vi "Autonomous Independent.vi"() -> ()   [LabVIEW 2020]
doc: "This VI is called when autonomous begins, and will automatically be terminated when autonomous ends. You can carry out timed or sensor driven robot movement independently without needing to return to the caller."
uses:
  <vilib>/Rock Robotics/WPI/RobotDrive/WPI_RobotDriveArcadeDrive_Standard(NoSaturation).vi
  <vilib>/Rock Robotics/Network Tables/NT Write Numeric Array.vi
  <vilib>/Rock Robotics/Network Tables/NT Read String.vi
panel:
  in  "Array for intake":cluster{"Delay (sec)":dbl, "On or Off":bool}[](array[cluster])
  out "Current Movement, for debugging":T1 {"Y Joystick Value" scale=1.0..-1.0; "X Joystick Value" scale=-1.0..1.0}
  in  "Array of robot movements":T2(array[cluster])=[{"X Joystick Value"=0.39393939393939403, "Y Joystick Value"=0.0, "Delay (sec)"=1.0, "Movement Name"="turn"}, {"X Joystick Value"=-0.3737373737373737, "Y Joystick Value"=0.0, "Delay (sec)"=1.0, "Movement Name"="turn back"}] {"Y Joystick Value" scale=1.0..-1.0; "X Joystick Value" scale=-1.0..1.0}
  # "Be sure to right-click and choose Data Operations>>Make Current Value default if you want to save the array values with the VI"
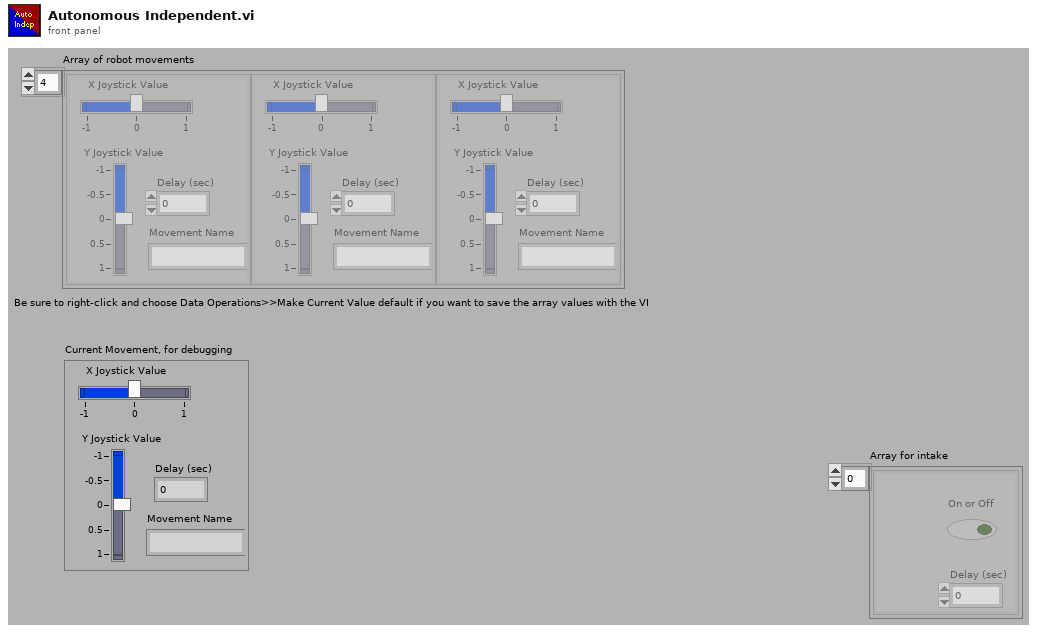
[diagram p1: front panel]
types:
  T1 = cluster{"X Joystick Value":dbl, "Y Joystick Value":dbl, "Delay (sec)":dbl, "Movement Name":string}
  T2 = cluster{"X Joystick Value":dbl, "Y Joystick Value":dbl, "Delay (sec)":dbl, "Movement Name":string}[]
  T3 = typedef "WPI_JoystickDevRef.ctl" = cluster{"Device":T4}
  T4 = typedef "WPI_JoystickDeviceEnum.ctl" = enum16{"USB 0", "USB 1", "USB 2", "USB 3", "USB 4", "USB 5"}
  T5 = typedef "WPI_MotorControlDeviceRef.ctl" = cluster{"DeviceStatus":errorcluster, "Type":T6, "PWM":cluster{"PWM Channel":T7, "DeadBand":T8}, "CAN":cluster{"Device Number":u8, "SetOutput VI Ref":variant, "GetOutput VI Ref":variant, "Enable VI Ref":variant, "Disable VI Ref":variant, "Data":variant}, "Invert":bool, "DIO PWM":cluster{"PWM \"Enable\" Channel":T7, "DIOChannel":T9, "PWM Rate":dbl}}
  T6 = typedef "WPI_MotorControlType.ctl" = enum16{"PWM", "CAN", "DIO PWM"}
  T7 = typedef "FPGA_DIOPWMChannel.ctl" = enum8{"PWM 0", "PWM 1", "PWM 2", "PWM 3", "PWM 4", "PWM 5", "PWM 6", "PWM 7", "PWM 8", "PWM 9", "PWM MXP 0", "PWM MXP 1", "PWM MXP 2", "PWM MXP 3", "PWM MXP 4", "PWM MXP 5", "PWM MXP 6", "PWM MXP 7", "PWM MXP 8", "PWM MXP 9", "Invalid"}
  T8 = typedef "WPI_PWMDeadband.ctl" = cluster{"Name":string, "maxPositivePwm":i32, "minPositivePwm":i32, "centerPwm":i32, "maxNegativePwm":i32, "minNegativePwm":i32, "angularRange":u16}
  T9 = typedef "FPGA_DIOChannel.ctl" = enum8{"DIO 0", "DIO 1", "DIO 2", "DIO 3", "DIO 4", "DIO 5", "DIO 6", "DIO 7", "DIO 8", "DIO 9", "DIO MXP 0", "DIO MXP 1", "DIO MXP 2", "DIO MXP 3", "DIO MXP 4", "DIO MXP 5", "DIO MXP 6", "DIO MXP 7", "DIO MXP 8", "DIO MXP 9", "DIO MXP 10", "DIO MXP 11", "DIO MXP 12", "DIO MXP 13", "DIO MXP 14", "DIO MXP 15", "SPI Port CS1", "SPI Port CS2", "SPI Port CS3", "SPI Port MISO", "SPI Port MOSI", "Invalid"}
  T10 = typedef "WPI_RobotDriveDevRef.ctl" = cluster{"DevStatus":errorcluster, "Motors[]":T5[], "Square Inputs":bool, "Max Output":dbl}
  T11 = cluster{"Yaw":dbl, "Roll":dbl, "Pitch":dbl, "Heading":dbl, "Fused Heading":dbl}
  T12 = typedef "Color Sensor V3 DevRef.ctl" = cluster{"I2CDevRef":T13}
  T13 = typedef "WPI_I2CDevRef.ctl" = cluster{"DevStatus":errorcluster, "Device Address":u8, "Handle":i32, "I2C Bus":T14}
  T14 = typedef "i2c_bus.ctl" = enum16{"I2C On-Board", "I2C MXP", "Invalid"}
  T15 = typedef "WPI_SwitchDevRef.ctl" = cluster{"DevStatus":errorcluster, "DIO Channel":T9, "CntIndex":T16, "Normally Closed":bool}
  T16 = typedef "FPGA_CounterCtrSystemIndex.ctl" = enum8{"Ctr 0", "Ctr 1", "Ctr 2", "Ctr 3", "Ctr 4", "Ctr 5", "Ctr 6", "Ctr 7", "Invalid"}
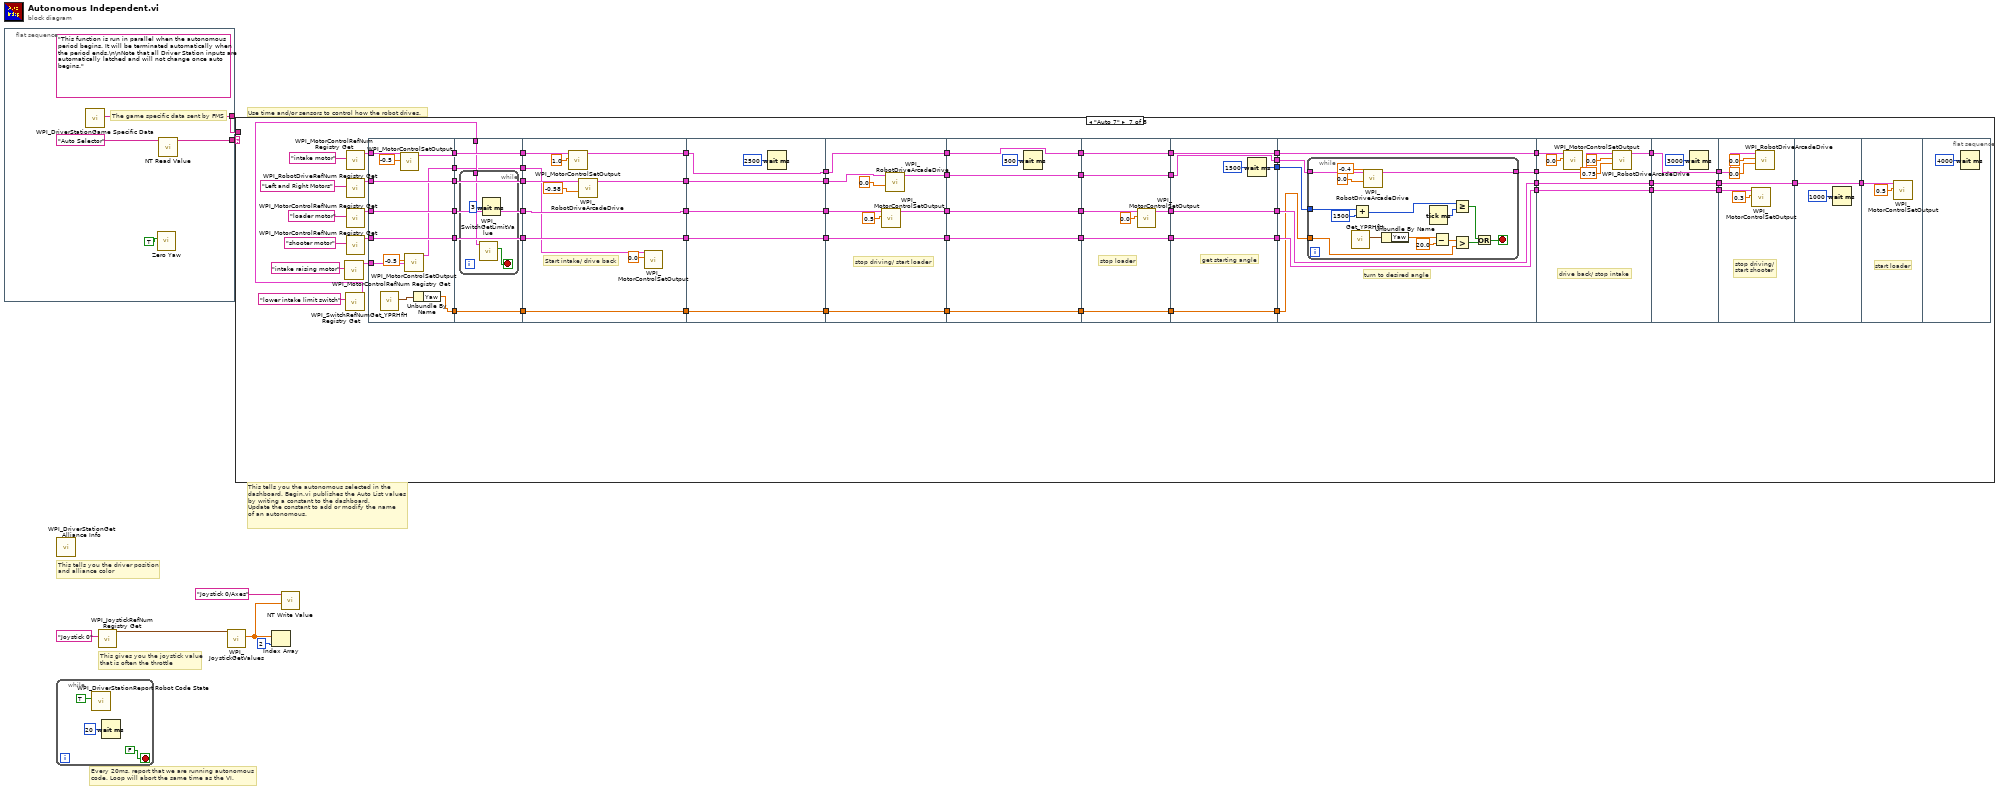
[diagram p0: block diagram]
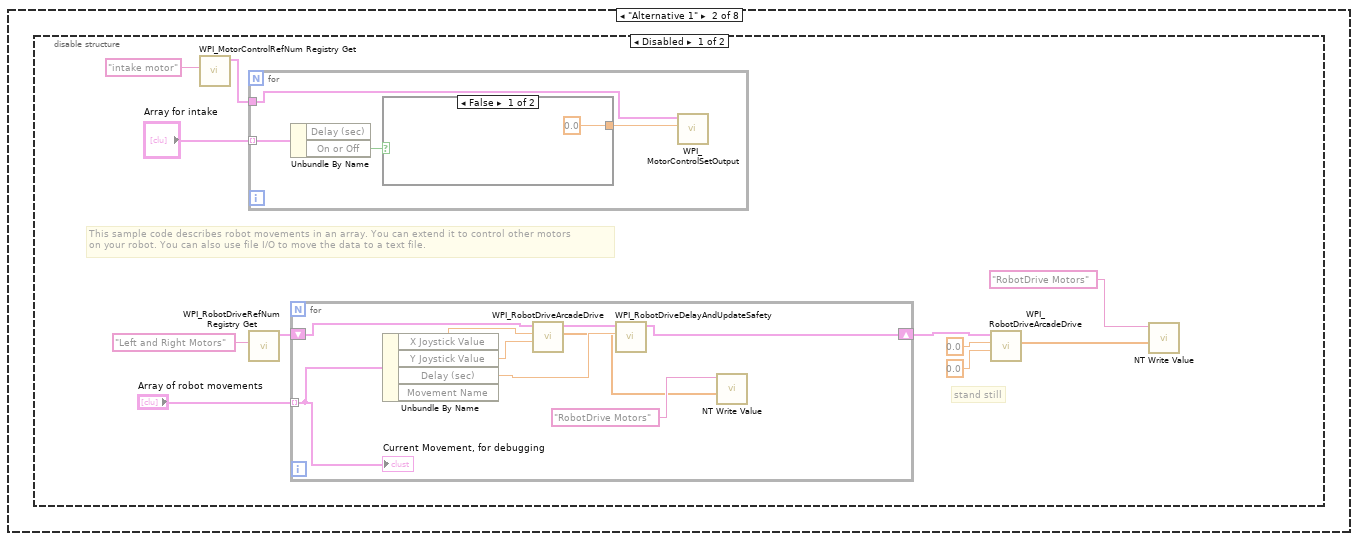
[diagram p3: hidden frame]
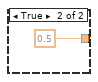
[diagram p4: hidden frame]
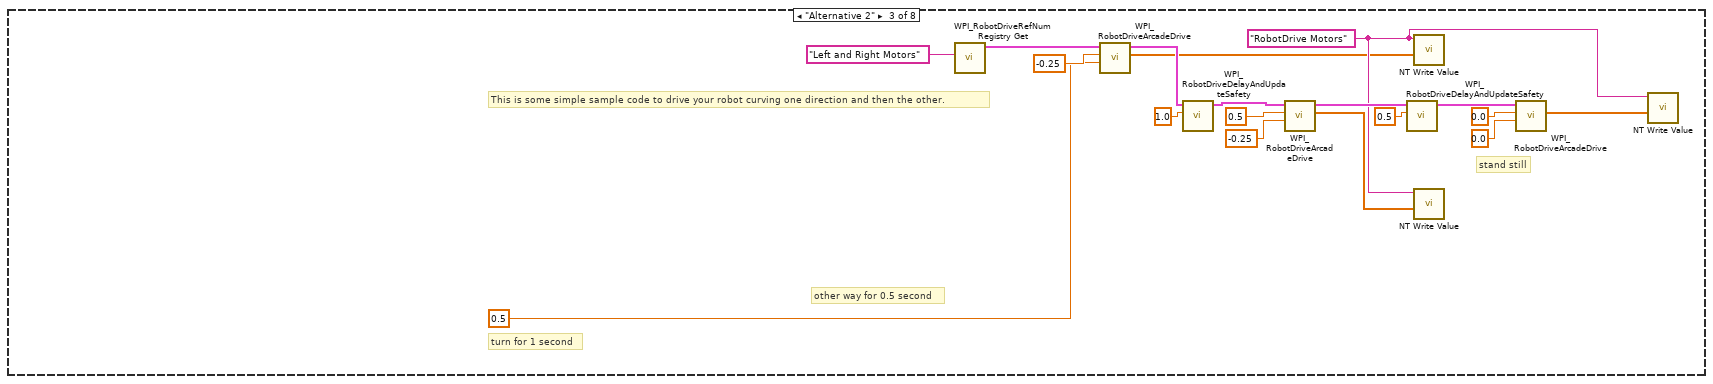
[diagram p6: hidden frame]
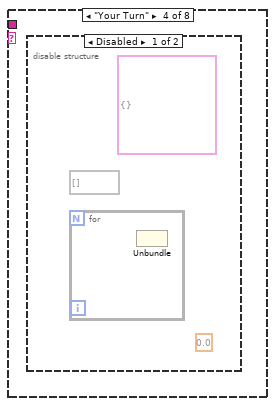
[diagram p7: hidden frame]
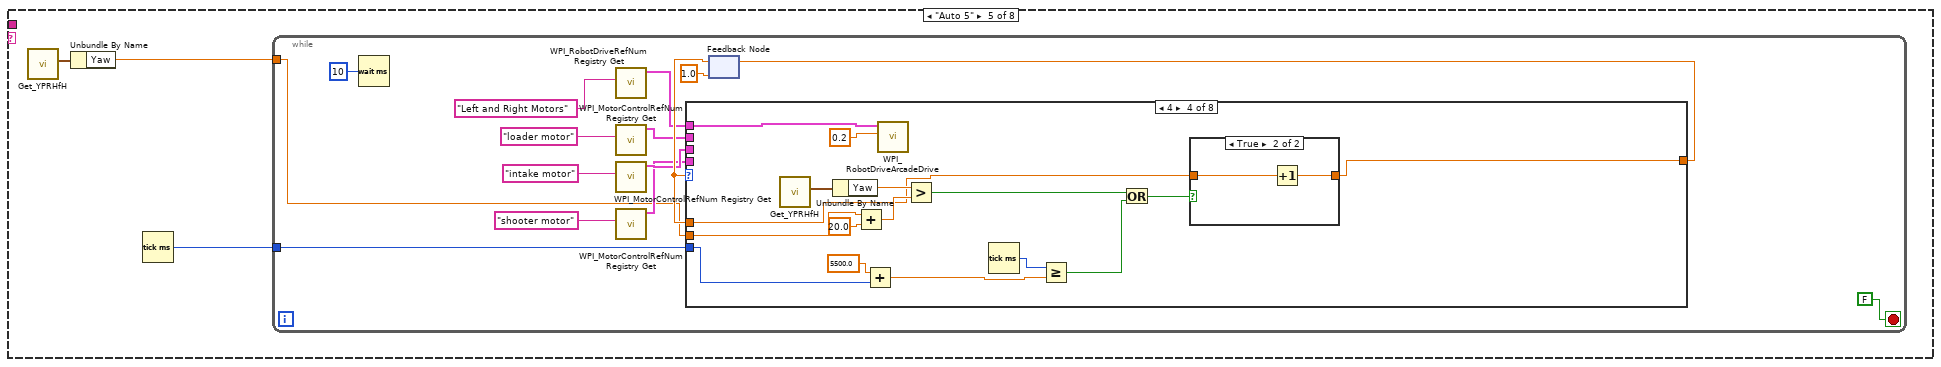
[diagram p9: hidden frame]
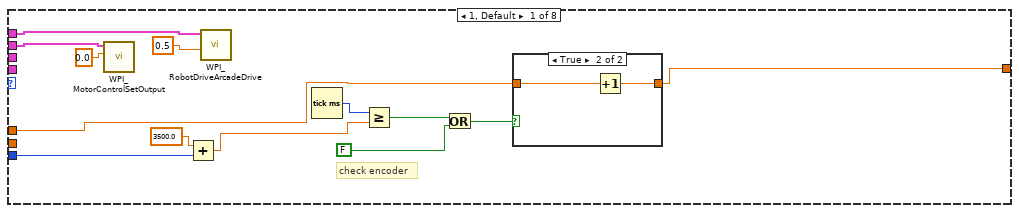
[diagram p10: hidden frame]
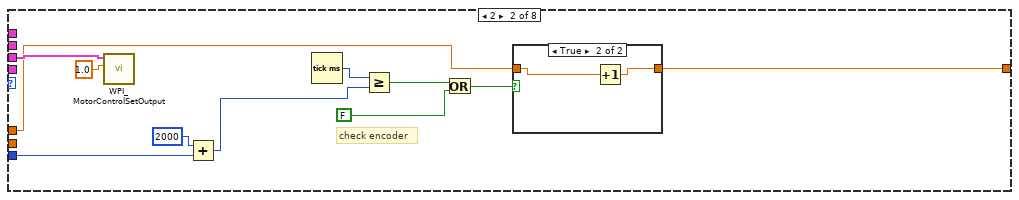
[diagram p12: hidden frame]
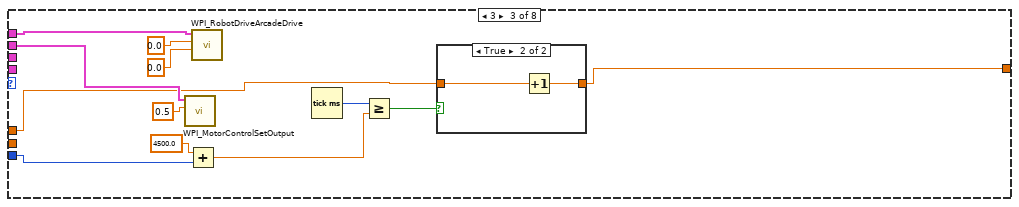
[diagram p14: hidden frame]
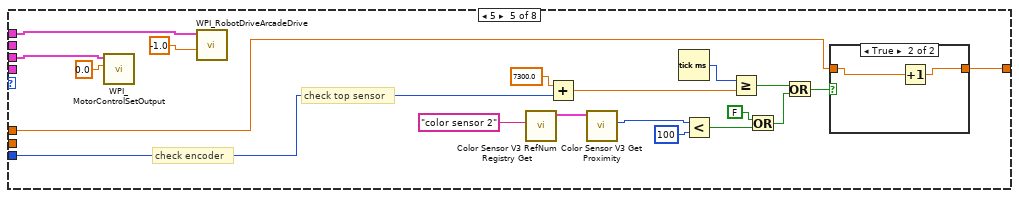
[diagram p17: hidden frame]
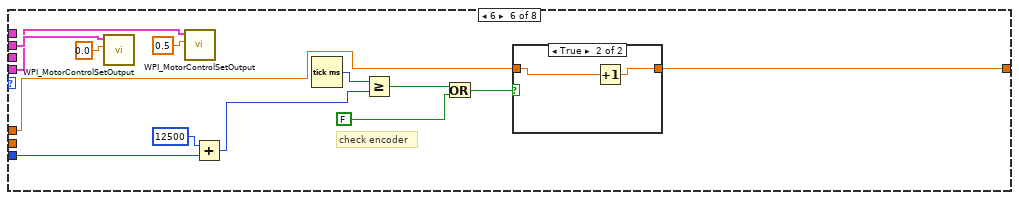
[diagram p19: hidden frame]
diagram:
  # "This tells you the autonomous selected in the \ndashboard. Begin.vi publishes the Auto List values\nby writing a constant to the dashboard.\nUpdate the constant to add or modify the name\nof an autonomous."
  # "Every 20ms, report that we are running autonomous\ncode. Loop will abort the same time as the VI."
  # "This gives you the joystick value\nthat is often the throttle"
  # "Use time and/or sensors to control how the robot drives."
  # "This tells you the driver position\nand alliance color"
  n1 = flat-sequence {
    tunnel: [w10] -> w4
    tunnel: [w9] -> w1
    frame #0 {
      (unwired) "This function is run in parallel when the autonomous period begins. It will be terminated automatically when the period ends.\n\nNote that all Driver Station inputs are automatically latched and will not change once auto begins."
      # "The game specific data sent by FMS"
      n2 = call <vilib>:"WPI_DriverStationGame Specific Data.vi"() -> ("Game Specific Data"=w9:string)  [unwired: 11 in]
      n3 = call <vilib>:"Zero Yaw.vi"("Zero"=TRUE) -> ()  [unwired: 11 in]
      n4 = call-poly <vilib>:"NT Read Value.vi"("Name"="Auto Selector") -> ("String"=w10:string)  [unwired: 9 in, 1 out]
    }
  }
  n5 = call <vilib>:"WPI_DriverStationGet Alliance Info.vi"() -> ()  [unwired: 12 out]
  n6 = while {
    stop <- FALSE stop-if-true
    n7 = call <vilib>:"WPI_DriverStationReport Robot Code State.vi"("Autonomous"=TRUE) -> ()  [unwired: 10 in, 1 out]
    n8 = Wait (ms)(milliseconds to wait=u32 20) -> ()  [unwired: 1 out]
  }
  n9 = call <vilib>:"WPI_JoystickRefNum Registry Get.vi"("refnum name"="Joystick 0") -> ("JoystickDevRef"=w6:T3)  [unwired: 1 in, 9 out]
  n10 = call <vilib>:"WPI_JoystickGetValues.vi"("JoystickDevRef"=w6) -> ("Axes"=w3:dbl[])  [unwired: 6 in, 4 out]
  n11 = case shown="\"Auto 7\"" w4 {
    tunnel: w1 -> [_ _ _ _ _ _ _ _]
    frame Default {
      # "You can put your main auto here, or you can right-click on the case and make any\nother frame be the default case."
      # "This is the frame that will execute if no selection is made, or if it is not recognized"
    }
    frame "Alternative 1" {
      n12 = disable-structure shown="Disabled" {
        frame Disabled {
          # "stand still"
          # "This sample code describes robot movements in an array. You can extend it to control other motors\non your robot. You can also use file I/O to move the data to a text file."
          n13 = call <vilib>:"WPI_MotorControlRefNum Registry Get.vi"("refnum name"="intake motor") -> ("MotorControlDevRef"=w15:T5)  [unwired: 9 in, 1 out]
          n14 = for {
            tunnel: "Array for intake" -> [w29] mode=indexing
            tunnel: w15 -> [w26]
            n15 = Unbundle By Name(w29) -> ("On or Off"=w28:bool)  [unwired: 1 out]
            n16 = case shown="False" w28 {
              tunnel: [0.0 ("Output") 0.5 ("Output")] -> w27
              frame False {
              }
              frame True {
              }
            }
            n17 = call <vilib>:"WPI_MotorControlSetOutput.vi"("Output"=w27, "MotorControlDevRef"=w26) -> ()  [unwired: 7 in, 3 out]
          }
          n18 = call <vilib>:"WPI_RobotDriveRefNum Registry Get.vi"("refnum name"="Left and Right Motors") -> ("RobotDriveDevRef"=w24:T10)  [unwired: 1 in, 9 out]
          n19 = for {
            shift-right: [w38] -> w19
            shift-left: w24 -> [w39]
            tunnel: "Array of robot movements" -> [w34] mode=indexing
            n20 = Unbundle By Name(w34) -> ("X Joystick Value"=w37:dbl, "Y Joystick Value"=w36:dbl, "Delay (sec)"=w35:dbl)  [unwired: 1 out]
            n21 = call-poly <vilib>:"WPI_RobotDriveArcadeDrive.vi"("Y axis value"=w36, "X axis value"=w37, "RobotDriveDevRef"=w39) -> ("Motor Values"=w32:dbl[], "RobotDriveDevRef"=w40:T10)  [unwired: 1 in, 6 out]
            n22 = call <vilib>:"WPI_RobotDriveDelayAndUpdateSafety.vi"("Delay (s)"=w35, "RobotDriveDevRef"=w40) -> ("RobotDriveDevRef 2"=w38:T10)  [unwired: 8 in, 1 out]
            n23 = call-poly <vilib>:"NT Write Value.vi"("Numeric Array"=w32, "Name"="RobotDrive Motors") -> ()  [unwired: 9 in, 1 out]
            "Current Movement, for debugging" <- w34
          }
          n24 = call-poly <vilib>:"WPI_RobotDriveArcadeDrive.vi"("Y axis value"=0.0 ("X axis value"), "X axis value"=0.0, "RobotDriveDevRef"=w19) -> ("Motor Values"=w22:dbl[])  [unwired: 1 in, 7 out]
          n25 = call-poly <vilib>:"NT Write Value.vi"("Numeric Array"=w22, "Name"="RobotDrive Motors") -> ()  [unwired: 9 in, 1 out]
        }
        frame Enabled {
        }
      }
    }
    frame "Alternative 2" {
      w42 = "RobotDrive Motors" ("Name")
      # "This is some simple sample code to drive your robot curving one direction and then the other."
      # "stand still"
      # "other way for 0.5 second"
      # "turn for 1 second"
      n26 = call <vilib>:"WPI_RobotDriveRefNum Registry Get.vi"("refnum name"="Left and Right Motors") -> ("RobotDriveDevRef"=w58:T10)  [unwired: 1 in, 9 out]
      n27 = call-poly <vilib>:"WPI_RobotDriveArcadeDrive.vi"("Y axis value"=0.5 ("X axis value"), "X axis value"=-0.25, "RobotDriveDevRef"=w58) -> ("Motor Values"=w41:dbl[], "RobotDriveDevRef"=w51:T10)  [unwired: 1 in, 6 out]
      n28 = call <vilib>:"WPI_RobotDriveDelayAndUpdateSafety.vi"("Delay (s)"=1.0, "RobotDriveDevRef"=w51) -> ("RobotDriveDevRef 2"=w52:T10)  [unwired: 8 in, 1 out]
      n29 = call-poly <vilib>:"WPI_RobotDriveArcadeDrive.vi"("Y axis value"=-0.25 ("X axis value"), "X axis value"=0.5, "RobotDriveDevRef"=w52) -> ("Motor Values"=w43:dbl[], "RobotDriveDevRef"=w53:T10)  [unwired: 1 in, 6 out]
      n30 = call <vilib>:"WPI_RobotDriveDelayAndUpdateSafety.vi"("Delay (s)"=0.5, "RobotDriveDevRef"=w53) -> ("RobotDriveDevRef 2"=w54:T10)  [unwired: 8 in, 1 out]
      n31 = call-poly <vilib>:"NT Write Value.vi"("Numeric Array"=w41, "Name"=w42) -> ()  [unwired: 9 in, 1 out]
      n32 = call-poly <vilib>:"NT Write Value.vi"("Numeric Array"=w43, "Name"=w42) -> ()  [unwired: 9 in, 1 out]
      n33 = call-poly <vilib>:"WPI_RobotDriveArcadeDrive.vi"("Y axis value"=0.0 ("X axis value"), "X axis value"=0.0, "RobotDriveDevRef"=w54) -> ("Motor Values"=w44:dbl[])  [unwired: 1 in, 7 out]
      n34 = call-poly <vilib>:"NT Write Value.vi"("Numeric Array"=w44, "Name"=w42) -> ()  [unwired: 9 in, 1 out]
    }
    frame "Your Turn" {
      n35 = disable-structure shown="Disabled" {
        frame Disabled {
          (unwired) cluster{} {}
          (unwired) 0.0
          (unwired) void[] []
          n36 = for {
            n37 = Unbundle() -> ()  [unwired: 1 in, 2 out]
          }
        }
        frame Enabled {
        }
      }
    }
    frame "Auto 5" {
      n38 = call <vilib>:"Get_YPRHfH.vi"() -> ("YRPHfH"=w60:T11)  [unwired: 11 in]
      n39 = Unbundle By Name(w60) -> ("Yaw"=w59:dbl)
      n40 = Tick Count (ms)() -> (millisecond timer value=w61:u32)
      n41 = while {
        tunnel: w61 -> [w63]
        tunnel: w59 -> [w62]
        stop <- FALSE stop-if-true
        n42 = Wait (ms)(milliseconds to wait=u32 10) -> ()  [unwired: 1 out]
        n43 = call <vilib>:"WPI_RobotDriveRefNum Registry Get.vi"("refnum name"="Left and Right Motors") -> ("RobotDriveDevRef"=w70:T10)  [unwired: 9 in, 1 out]
        n44 = call <vilib>:"WPI_MotorControlRefNum Registry Get.vi"("refnum name"="loader motor") -> ("MotorControlDevRef"=w68:T5)  [unwired: 9 in, 1 out]
        n45 = call <vilib>:"WPI_MotorControlRefNum Registry Get.vi"("refnum name"="intake motor") -> ("MotorControlDevRef"=w72:T5)  [unwired: 9 in, 1 out]
        n46 = call <vilib>:"WPI_MotorControlRefNum Registry Get.vi"("refnum name"="shooter motor") -> ("MotorControlDevRef"=w66:T5)  [unwired: 9 in, 1 out]
        n47 = feedback #1(1.0) -> (w74:dbl)
        n48 = case shown="4" w74 {
          tunnel: w74 -> [w89 w101 w112 w125 w156 w170 w184 w194]
          tunnel: [w88 w100 w113 w124 w157 w171 w185 w194] -> w76
          tunnel: w72 -> [_ w102 _ _ w151 _ _ _]
          tunnel: w70 -> [w84 _ w118 w126 w159 _ w188 _]
          tunnel: w68 -> [w78 _ w115 _ _ w175 _ w193]
          tunnel: w66 -> [_ _ _ _ _ w163 _ _]
          tunnel: w63 -> [w79 w95 w107 w123 w146 w166 w180 _]
          tunnel: w62 -> [_ _ _ w122 _ _ _ _]
          frame 1, Default {
            # "check encoder"
            n49 = call <vilib>:"WPI_MotorControlSetOutput.vi"("Output"=0.0, "MotorControlDevRef"=w78) -> ()  [unwired: 7 in, 3 out]
            n50 = Add(x=3500.0 ("y"), y=w79) -> (x+y=w81:dbl)
            n51 = call-poly <vilib>:"WPI_RobotDriveArcadeDrive.vi"("Y axis value"=0.5, "RobotDriveDevRef"=w84) -> ()  [unwired: 7 in, 3 out]
            n52 = Tick Count (ms)() -> (millisecond timer value=w82:u32)
            n53 = Greater Or Equal?(x=w82, y=w81) -> (x >= y?=w86:bool)
            n54 = Or(x=w86, y=FALSE) -> (x .or. y?=w87:bool)
            n55 = case shown="True" w87 {
              tunnel: w89 -> [w90 w91]
              tunnel: [w90 w92] -> w88
              frame False {
              }
              frame True {
                n56 = Increment(x=w91) -> (x+1=w92:dbl)
              }
            }
          }
          frame 2 {
            # "check encoder"
            n57 = call <vilib>:"WPI_MotorControlSetOutput.vi"("Output"=1.0, "MotorControlDevRef"=w102) -> ()  [unwired: 7 in, 3 out]
            n58 = Add(x=u32 2000, y=w95) -> (x+y=w96:u32)
            n59 = Tick Count (ms)() -> (millisecond timer value=w93:u32)
            n60 = Greater Or Equal?(x=w93, y=w96) -> (x >= y?=w98:bool)
            n61 = Or(x=w98, y=FALSE) -> (x .or. y?=w99:bool)
            n62 = case shown="True" w99 {
              tunnel: w101 -> [w104 w106]
              tunnel: [w104 w105] -> w100
              frame False {
              }
              frame True {
                n63 = Increment(x=w106) -> (x+1=w105:dbl)
              }
            }
          }
          frame 3 {
            n64 = call <vilib>:"WPI_MotorControlSetOutput.vi"("Output"=0.5, "MotorControlDevRef"=w115) -> ()  [unwired: 7 in, 3 out]
            n65 = Add(x=4500.0, y=w107) -> (x+y=w109:dbl)
            n66 = call-poly <vilib>:"WPI_RobotDriveArcadeDrive.vi"("Y axis value"=0.0, "X axis value"=0.0, "RobotDriveDevRef"=w118) -> ()  [unwired: 6 in, 3 out]
            n67 = Tick Count (ms)() -> (millisecond timer value=w110:u32)
            n68 = Greater Or Equal?(x=w110, y=w109) -> (x >= y?=w111:bool)
            n69 = case shown="True" w111 {
              tunnel: [w119 w121] -> w113
              tunnel: w112 -> [w119 w120]
              frame False {
              }
              frame True {
                n70 = Increment(x=w120) -> (x+1=w121:dbl)
              }
            }
          }
          frame 4 {
            n71 = call <vilib>:"Get_YPRHfH.vi"() -> ("YRPHfH"=w131:T11)  [unwired: 11 in]
            n72 = Unbundle By Name(w131) -> ("Yaw"=w130:dbl)
            n73 = Add(x=w122, y=20.0) -> (x+y=w128:dbl)
            n74 = Add(x=5500.0, y=w123) -> (x+y=w136:dbl)
            n75 = call-poly <vilib>:"WPI_RobotDriveArcadeDrive.vi"("X axis value"=0.2, "RobotDriveDevRef"=w126) -> ()  [unwired: 7 in, 3 out]
            n76 = Greater?(x=w130, y=w128) -> (0:w129:bool)
            n77 = Tick Count (ms)() -> (millisecond timer value=w137:u32)
            n78 = Greater Or Equal?(x=w137, y=w136) -> (x >= y?=w133:bool)
            n79 = Or(x=w129, y=w133) -> (x .or. y?=w132:bool)
            n80 = case shown="True" w132 {
              tunnel: [w138 w140] -> w124
              tunnel: w125 -> [w138 w139]
              frame False {
              }
              frame True {
                n81 = Increment(x=w139) -> (x+1=w140:dbl)
              }
            }
          }
          frame 5 {
            # "check top sensor"
            # "check encoder"
            n82 = call <vilib>:"WPI_MotorControlSetOutput.vi"("Output"=0.0, "MotorControlDevRef"=w151) -> ()  [unwired: 7 in, 3 out]
            n83 = call-poly <vilib>:"WPI_RobotDriveArcadeDrive.vi"("Y axis value"=-1.0, "RobotDriveDevRef"=w159) -> ()  [unwired: 7 in, 3 out]
            n84 = call <vilib>:"Color Sensor V3 RefNum Registry Get.vi"("refnum name"="color sensor 2") -> ("ColorSensorDevRef"=w144:T12)  [unwired: 9 in, 1 out]
            n85 = Add(x=7300.0, y=w146) -> (x+y=w148:dbl)
            n86 = call <vilib>:"Color Sensor V3 Get Proximity.vi"("ColorSensorDevRef"=w144) -> ("Proximity"=w143:u16)  [unwired: 8 in, 2 out]
            n87 = Tick Count (ms)() -> (millisecond timer value=w149:u32)
            n88 = Less?(x=w143, y=u16 100) -> (x < y?=w141:bool)
            n89 = Greater Or Equal?(x=w149, y=w148) -> (x >= y?=w153:bool)
            n90 = Or(x=FALSE, y=w141) -> (x .or. y?=w154:bool)
            n91 = Or(x=w153, y=w154) -> (x .or. y?=w155:bool)
            n92 = case shown="True" w155 {
              tunnel: [w160 w162] -> w157
              tunnel: w156 -> [w160 w161]
              frame False {
              }
              frame True {
                n93 = Increment(x=w161) -> (x+1=w162:dbl)
              }
            }
          }
          frame 6 {
            # "check encoder"
            n94 = call <vilib>:"WPI_MotorControlSetOutput.vi"("Output"=0.0, "MotorControlDevRef"=w175) -> ()  [unwired: 7 in, 3 out]
            n95 = call <vilib>:"WPI_MotorControlSetOutput.vi"("Output"=0.5, "MotorControlDevRef"=w163) -> ()  [unwired: 7 in, 3 out]
            n96 = Add(x=u32 12500, y=w166) -> (x+y=w167:u32)
            n97 = Tick Count (ms)() -> (millisecond timer value=w168:u32)
            n98 = Greater Or Equal?(x=w168, y=w167) -> (x >= y?=w172:bool)
            n99 = Or(x=w172, y=FALSE) -> (x .or. y?=w173:bool)
            n100 = case shown="True" w173 {
              tunnel: [w176 w178] -> w171
              tunnel: w170 -> [w176 w177]
              frame False {
              }
              frame True {
                n101 = Increment(x=w177) -> (x+1=w178:dbl)
              }
            }
          }
          frame 7 {
            n102 = call-poly <vilib>:"WPI_RobotDriveArcadeDrive.vi"("Y axis value"=0.0, "X axis value"=0.0, "RobotDriveDevRef"=w188) -> ()  [unwired: 6 in, 3 out]
            n103 = Add(x=u32 13000, y=w180) -> (x+y=w181:u32)
            n104 = Tick Count (ms)() -> (millisecond timer value=w182:u32)
            n105 = Greater Or Equal?(x=w182, y=w181) -> (x >= y?=w183:bool)
            n106 = case shown="True" w183 {
              tunnel: [w189 w191] -> w185
              tunnel: w184 -> [w189 w190]
              frame False {
              }
              frame True {
                n107 = Increment(x=w190) -> (x+1=w191:dbl)
              }
            }
          }
          frame 8 {
            n108 = call <vilib>:"WPI_MotorControlSetOutput.vi"("Output"=0.3, "MotorControlDevRef"=w193) -> ()  [unwired: 7 in, 3 out]
          }
        }
        n109 = feedback-in #1(w76) -> ()
      }
    }
    frame "Auto 6" {
      n110 = call <vilib>:"Get_YPRHfH.vi"() -> ("YRPHfH"=w196:T11)  [unwired: 11 in]
      n111 = Unbundle By Name(w196) -> ("Yaw"=w195:dbl)
      n112 = Tick Count (ms)() -> (millisecond timer value=w197:u32)
      n113 = while {
        tunnel: w197 -> [w199]
        tunnel: w195 -> [w198]
        stop <- FALSE stop-if-true
        n114 = Wait (ms)(milliseconds to wait=u32 10) -> ()  [unwired: 1 out]
        n115 = call <vilib>:"WPI_RobotDriveRefNum Registry Get.vi"("refnum name"="Left and Right Motors") -> ("RobotDriveDevRef"=w206:T10)  [unwired: 9 in, 1 out]
        n116 = call <vilib>:"WPI_MotorControlRefNum Registry Get.vi"("refnum name"="loader motor") -> ("MotorControlDevRef"=w204:T5)  [unwired: 9 in, 1 out]
        n117 = call <vilib>:"WPI_MotorControlRefNum Registry Get.vi"("refnum name"="intake motor") -> ("MotorControlDevRef"=w208:T5)  [unwired: 9 in, 1 out]
        n118 = call <vilib>:"WPI_MotorControlRefNum Registry Get.vi"("refnum name"="shooter motor") -> ("MotorControlDevRef"=w202:T5)  [unwired: 9 in, 1 out]
        n119 = feedback #2(1.0) -> (w210:dbl)
        n120 = case shown="6" w210 {
          tunnel: w210 -> [w225 w237 w248 w269 w292 w306 w320 w330]
          tunnel: [w224 w236 w249 w268 w293 w307 w321 w330] -> w212
          tunnel: w208 -> [_ w238 _ _ w287 _ _ _]
          tunnel: w206 -> [w220 _ w254 w264 w295 _ w324 _]
          tunnel: w204 -> [w214 _ w251 _ _ w311 _ w329]
          tunnel: w202 -> [_ _ _ _ _ w299 _ _]
          tunnel: w199 -> [w215 w231 w243 w270 w282 w302 w316 _]
          tunnel: w198 -> [_ _ _ w260 _ _ _ _]
          frame 1, Default {
            # "check encoder"
            n121 = call <vilib>:"WPI_MotorControlSetOutput.vi"("Output"=0.0, "MotorControlDevRef"=w214) -> ()  [unwired: 7 in, 3 out]
            n122 = Add(x=500.0 ("y"), y=w215) -> (x+y=w217:dbl)
            n123 = call-poly <vilib>:"WPI_RobotDriveArcadeDrive.vi"("Y axis value"=0.5, "RobotDriveDevRef"=w220) -> ()  [unwired: 7 in, 3 out]
            n124 = Tick Count (ms)() -> (millisecond timer value=w218:u32)
            n125 = Greater Or Equal?(x=w218, y=w217) -> (x >= y?=w222:bool)
            n126 = Or(x=w222, y=FALSE) -> (x .or. y?=w223:bool)
            n127 = case shown="True" w223 {
              tunnel: w225 -> [w226 w227]
              tunnel: [w226 w228] -> w224
              frame False {
              }
              frame True {
                n128 = Increment(x=w227) -> (x+1=w228:dbl)
              }
            }
          }
          frame 2 {
            # "check encoder"
            n129 = call <vilib>:"WPI_MotorControlSetOutput.vi"("Output"=1.0, "MotorControlDevRef"=w238) -> ()  [unwired: 7 in, 3 out]
            n130 = Add(x=u32 2000, y=w231) -> (x+y=w232:u32)
            n131 = Tick Count (ms)() -> (millisecond timer value=w229:u32)
            n132 = Greater Or Equal?(x=w229, y=w232) -> (x >= y?=w234:bool)
            n133 = Or(x=w234, y=FALSE) -> (x .or. y?=w235:bool)
            n134 = case shown="True" w235 {
              tunnel: w237 -> [w240 w242]
              tunnel: [w240 w241] -> w236
              frame False {
              }
              frame True {
                n135 = Increment(x=w242) -> (x+1=w241:dbl)
              }
            }
          }
          frame 3 {
            n136 = call <vilib>:"WPI_MotorControlSetOutput.vi"("Output"=0.5, "MotorControlDevRef"=w251) -> ()  [unwired: 7 in, 3 out]
            n137 = Add(x=4500.0, y=w243) -> (x+y=w245:dbl)
            n138 = call-poly <vilib>:"WPI_RobotDriveArcadeDrive.vi"("Y axis value"=0.0, "X axis value"=0.0, "RobotDriveDevRef"=w254) -> ()  [unwired: 6 in, 3 out]
            n139 = Tick Count (ms)() -> (millisecond timer value=w246:u32)
            n140 = Greater Or Equal?(x=w246, y=w245) -> (x >= y?=w247:bool)
            n141 = case shown="True" w247 {
              tunnel: [w255 w257] -> w249
              tunnel: w248 -> [w255 w256]
              frame False {
              }
              frame True {
                n142 = Increment(x=w256) -> (x+1=w257:dbl)
              }
            }
          }
          frame 4 {
            n143 = call <vilib>:"Get_YPRHfH.vi"() -> ("YRPHfH"=w263:T11)  [unwired: 11 in]
            n144 = Unbundle By Name(w263) -> ("Yaw"=w262:dbl)
            n145 = Add(x=w260, y=-20.0) -> (x+y=w259:dbl)
            n146 = Add(x=5500.0, y=w270) -> (x+y=w272:dbl)
            n147 = call-poly <vilib>:"WPI_RobotDriveArcadeDrive.vi"("X axis value"=0.2, "RobotDriveDevRef"=w264) -> ()  [unwired: 7 in, 3 out]
            n148 = Greater?(x=w262, y=w259) -> (0:w261:bool)
            n149 = Tick Count (ms)() -> (millisecond timer value=w273:u32)
            n150 = Greater Or Equal?(x=w273, y=w272) -> (x >= y?=w266:bool)
            n151 = Or(x=w261, y=w266) -> (x .or. y?=w265:bool)
            n152 = case shown="True" w265 {
              tunnel: [w274 w276] -> w268
              tunnel: w269 -> [w274 w275]
              frame False {
              }
              frame True {
                n153 = Increment(x=w275) -> (x+1=w276:dbl)
              }
            }
          }
          frame 5 {
            # "check top sensor"
            # "check encoder"
            n154 = call <vilib>:"WPI_MotorControlSetOutput.vi"("Output"=0.0, "MotorControlDevRef"=w287) -> ()  [unwired: 7 in, 3 out]
            n155 = call-poly <vilib>:"WPI_RobotDriveArcadeDrive.vi"("Y axis value"=-1.0, "RobotDriveDevRef"=w295) -> ()  [unwired: 7 in, 3 out]
            n156 = call <vilib>:"Color Sensor V3 RefNum Registry Get.vi"("refnum name"="color sensor 2") -> ("ColorSensorDevRef"=w280:T12)  [unwired: 9 in, 1 out]
            n157 = Add(x=7300.0, y=w282) -> (x+y=w284:dbl)
            n158 = call <vilib>:"Color Sensor V3 Get Proximity.vi"("ColorSensorDevRef"=w280) -> ("Proximity"=w279:u16)  [unwired: 8 in, 2 out]
            n159 = Tick Count (ms)() -> (millisecond timer value=w285:u32)
            n160 = Less?(x=w279, y=u16 100) -> (x < y?=w277:bool)
            n161 = Greater Or Equal?(x=w285, y=w284) -> (x >= y?=w289:bool)
            n162 = Or(x=FALSE, y=w277) -> (x .or. y?=w290:bool)
            n163 = Or(x=w289, y=w290) -> (x .or. y?=w291:bool)
            n164 = case shown="True" w291 {
              tunnel: [w296 w298] -> w293
              tunnel: w292 -> [w296 w297]
              frame False {
              }
              frame True {
                n165 = Increment(x=w297) -> (x+1=w298:dbl)
              }
            }
          }
          frame 6 {
            # "check encoder"
            n166 = call <vilib>:"WPI_MotorControlSetOutput.vi"("Output"=0.0, "MotorControlDevRef"=w311) -> ()  [unwired: 7 in, 3 out]
            n167 = call <vilib>:"WPI_MotorControlSetOutput.vi"("Output"=0.5, "MotorControlDevRef"=w299) -> ()  [unwired: 7 in, 3 out]
            n168 = Add(x=u32 12500, y=w302) -> (x+y=w303:u32)
            n169 = Tick Count (ms)() -> (millisecond timer value=w304:u32)
            n170 = Greater Or Equal?(x=w304, y=w303) -> (x >= y?=w308:bool)
            n171 = Or(x=w308, y=FALSE) -> (x .or. y?=w309:bool)
            n172 = case shown="True" w309 {
              tunnel: [w312 w314] -> w307
              tunnel: w306 -> [w312 w313]
              frame False {
              }
              frame True {
                n173 = Increment(x=w313) -> (x+1=w314:dbl)
              }
            }
          }
          frame 7 {
            n174 = call-poly <vilib>:"WPI_RobotDriveArcadeDrive.vi"("Y axis value"=0.0, "X axis value"=0.0, "RobotDriveDevRef"=w324) -> ()  [unwired: 6 in, 3 out]
            n175 = Add(x=u32 13000, y=w316) -> (x+y=w317:u32)
            n176 = Tick Count (ms)() -> (millisecond timer value=w318:u32)
            n177 = Greater Or Equal?(x=w318, y=w317) -> (x >= y?=w319:bool)
            n178 = case shown="True" w319 {
              tunnel: [w325 w327] -> w321
              tunnel: w320 -> [w325 w326]
              frame False {
              }
              frame True {
                n179 = Increment(x=w326) -> (x+1=w327:dbl)
              }
            }
          }
          frame 8 {
            n180 = call <vilib>:"WPI_MotorControlSetOutput.vi"("Output"=0.3, "MotorControlDevRef"=w329) -> ()  [unwired: 7 in, 3 out]
          }
        }
        n181 = feedback-in #2(w212) -> ()
      }
    }
    frame "Auto 7" {
      n182 = call <vilib>:"WPI_MotorControlRefNum Registry Get.vi"("refnum name"="intake raising motor") -> ("MotorControlDevRef"=w343:T5)  [unwired: 9 in, 1 out]
      n183 = call <vilib>:"WPI_SwitchRefNum Registry Get.vi"("refnum name"="lower intake limit switch") -> ("SwitchDevRef"=w341:T15)  [unwired: 9 in, 1 out]
      n184 = call <vilib>:"WPI_MotorControlRefNum Registry Get.vi"("refnum name"="intake motor") -> ("MotorControlDevRef"=w392:T5)  [unwired: 9 in, 1 out]
      n185 = call <vilib>:"WPI_RobotDriveRefNum Registry Get.vi"("refnum name"="Left and Right Motors") -> ("RobotDriveDevRef"=w393:T10)  [unwired: 9 in, 1 out]
      n186 = call <vilib>:"WPI_MotorControlRefNum Registry Get.vi"("refnum name"="loader motor") -> ("MotorControlDevRef"=w387:T5)  [unwired: 9 in, 1 out]
      n187 = call <vilib>:"WPI_MotorControlRefNum Registry Get.vi"("refnum name"="shooter motor") -> ("MotorControlDevRef"=w369:T5)  [unwired: 9 in, 1 out]
      n188 = flat-sequence {
        tunnel: w369 -> [w406]
        tunnel: w387 -> [w407]
        tunnel: w392 -> [w405]
        tunnel: w393 -> [w408]
        tunnel: [w408] -> w352
        tunnel: [w404] -> w350
        tunnel: [w407] -> w348
        tunnel: [w406] -> w346
        tunnel: w343 -> [w402]
        tunnel: [w400] -> w339
        tunnel: [w398] -> w338
        tunnel: w352 -> [w415]
        tunnel: [w415] -> w351
        tunnel: w350 -> [w414]
        tunnel: [w414] -> w349
        tunnel: w348 -> [w413]
        tunnel: [w413] -> w347
        tunnel: w346 -> [w412]
        tunnel: [w412] -> w345
        tunnel: w341 -> [w411]
        tunnel: [w410] -> w340
        tunnel: w339 -> [w410]
        tunnel: w338 -> [w409]
        tunnel: [w409] -> w331
        tunnel: [w425] -> w390
        tunnel: [w424] -> w388
        tunnel: [w423] -> w372
        tunnel: [w422] -> w360
        tunnel: w351 -> [w429]
        tunnel: w349 -> [w427]
        tunnel: w347 -> [w424]
        tunnel: w345 -> [w422]
        tunnel: w340 -> [w421]
        tunnel: [w419] -> w332
        tunnel: w331 -> [w419]
        tunnel: [w434] -> w391
        tunnel: w390 -> [w434]
        tunnel: [w433] -> w389
        tunnel: w388 -> [w433]
        tunnel: [w432] -> w373
        tunnel: w372 -> [w432]
        tunnel: [w431] -> w361
        tunnel: w360 -> [w431]
        tunnel: [w430] -> w333
        tunnel: w332 -> [w430]
        tunnel: w391 -> [w444]
        tunnel: w389 -> [w442]
        tunnel: [w440] -> w383
        tunnel: [w439] -> w382
        tunnel: [w438] -> w374
        tunnel: w373 -> [w438]
        tunnel: [w437] -> w362
        tunnel: w361 -> [w437]
        tunnel: [w436] -> w334
        tunnel: w333 -> [w436]
        tunnel: w383 -> [w450]
        tunnel: [w450] -> w381
        tunnel: [w448] -> w379
        tunnel: w382 -> [w448]
        tunnel: [w447] -> w375
        tunnel: w374 -> [w447]
        tunnel: [w446] -> w363
        tunnel: w362 -> [w446]
        tunnel: [w445] -> w335
        tunnel: w334 -> [w445]
        tunnel: w381 -> [w457]
        tunnel: [w457] -> w380
        tunnel: w379 -> [w455]
        tunnel: [w454] -> w376
        tunnel: w375 -> [w454]
        tunnel: [w453] -> w364
        tunnel: w363 -> [w453]
        tunnel: [w452] -> w353
        tunnel: [w451] -> w336
        tunnel: w335 -> [w451]
        tunnel: [w463] -> w386
        tunnel: w380 -> [w463]
        tunnel: [w462] -> w385
        tunnel: [w461] -> w377
        tunnel: w376 -> [w461]
        tunnel: [w460] -> w365
        tunnel: w364 -> [w460]
        tunnel: [w459] -> w354
        tunnel: w353 -> [w459]
        tunnel: [w458] -> w337
        tunnel: w336 -> [w458]
        tunnel: w386 -> [w471]
        tunnel: w385 -> [w470]
        tunnel: [w469] -> w384
        tunnel: [w468] -> w378
        tunnel: w377 -> [w468]
        tunnel: [w467] -> w366
        tunnel: w365 -> [w467]
        tunnel: [w466] -> w355
        tunnel: w354 -> [w466]
        tunnel: w337 -> [w465]
        tunnel: w384 -> [w495]
        tunnel: w378 -> [w492]
        tunnel: [w490] -> w370
        tunnel: [w489] -> w367
        tunnel: w366 -> [w489]
        tunnel: [w488] -> w356
        tunnel: w355 -> [w488]
        tunnel: [w498] -> w371
        tunnel: w370 -> [w498]
        tunnel: [w497] -> w368
        tunnel: w367 -> [w497]
        tunnel: [w496] -> w357
        tunnel: w356 -> [w496]
        tunnel: w371 -> [w505]
        tunnel: w368 -> [w502]
        tunnel: [w500] -> w358
        tunnel: w357 -> [w500]
        tunnel: [w506] -> w359
        tunnel: w358 -> [w506]
        tunnel: w359 -> [w509]
        frame #0 {
          n189 = call <vilib>:"Get_YPRHfH.vi"() -> ("YRPHfH"=w399:T11)  [unwired: 11 in]
          n190 = call <vilib>:"WPI_MotorControlSetOutput.vi"("Output"=-0.5, "MotorControlDevRef"=w405) -> ("MotorControlDevRef"=w404:T5)  [unwired: 7 in, 2 out]
          n191 = call <vilib>:"WPI_MotorControlSetOutput.vi"("Output"=-0.5, "MotorControlDevRef"=w402) -> ("MotorControlDevRef"=w400:T5)  [unwired: 7 in, 2 out]
          n192 = Unbundle By Name(w399) -> ("Yaw"=w398:dbl)
        }
        frame #1 {
          n193 = while {
            tunnel: w411 -> [w417]
            stop <- w418 stop-if-true
            n194 = call <vilib>:"WPI_SwitchGetLimitValue.vi"("SwitchDevRef"=w417) -> ("Switch Pressed"=w418:bool)  [unwired: 8 in, 2 out]
            n195 = Wait (ms)(milliseconds to wait=u32 3) -> ()  [unwired: 1 out]
          }
        }
        frame #2 {
          # "Start intake/ drive back"
          n196 = call <vilib>:"WPI_MotorControlSetOutput.vi"("Output"=1.0, "MotorControlDevRef"=w427) -> ("MotorControlDevRef"=w423:T5)  [unwired: 7 in, 2 out]
          n197 = call-poly <vilib>:"WPI_RobotDriveArcadeDrive.vi"("Y axis value"=-0.58, "RobotDriveDevRef"=w429) -> ("RobotDriveDevRef"=w425:T10)  [unwired: 7 in, 2 out]
          n198 = call <vilib>:"WPI_MotorControlSetOutput.vi"("Output"=0.0, "MotorControlDevRef"=w421) -> ()  [unwired: 7 in, 3 out]
        }
        frame #3 {
          n199 = Wait (ms)(milliseconds to wait=u32 2500) -> ()  [unwired: 1 out]
        }
        frame #4 {
          # "stop driving/ start loader"
          n200 = call <vilib>:"WPI_MotorControlSetOutput.vi"("Output"=0.5, "MotorControlDevRef"=w442) -> ("MotorControlDevRef"=w439:T5)  [unwired: 7 in, 2 out]
          n201 = call-poly <vilib>:"WPI_RobotDriveArcadeDrive.vi"("Y axis value"=0.0, "RobotDriveDevRef"=w444) -> ("RobotDriveDevRef"=w440:T10)  [unwired: 7 in, 2 out]
        }
        frame #5 {
          n202 = Wait (ms)(milliseconds to wait=u32 500) -> ()  [unwired: 1 out]
        }
        frame #6 {
          # "stop loader"
          n203 = call <vilib>:"WPI_MotorControlSetOutput.vi"("Output"=0.0, "MotorControlDevRef"=w455) -> ("MotorControlDevRef"=w452:T5)  [unwired: 7 in, 2 out]
        }
        frame #7 {
          # "get starting angle"
          n204 = Wait (ms)(milliseconds to wait=u32 1500) -> (millisecond timer value=w462:u32)
        }
        frame #8 {
          # "turn to desired angle"
          n205 = while {
            tunnel: w465 -> [w486]
            tunnel: w471 -> [w482]
            tunnel: w470 -> [w475]
            tunnel: [w473] -> w469
            stop <- w479 stop-if-true
            n206 = call <vilib>:"Get_YPRHfH.vi"() -> ("YRPHfH"=w487:T11)  [unwired: 11 in]
            n207 = Add(x=w475, y=u32 1500) -> (x+y=w476:u32)
            n208 = call-poly <vilib>:"WPI_RobotDriveArcadeDrive.vi"("Y axis value"=0.0, "X axis value"=-0.4, "RobotDriveDevRef"=w482) -> ("RobotDriveDevRef"=w473:T10)  [unwired: 6 in, 2 out]
            n209 = Unbundle By Name(w487) -> ("Yaw"=w483:dbl)
            n210 = Tick Count (ms)() -> (millisecond timer value=w474:u32)
            n211 = Subtract(x=w483, y=20.0) -> (x-y=w485:dbl)
            n212 = Greater Or Equal?(x=w476, y=w474) -> (x >= y?=w477:bool)
            n213 = Greater?(x=w485, y=w486) -> (0:w480:bool)
            n214 = Or(x=w477, y=w480) -> (x .or. y?=w479:bool)
          }
        }
        frame #9 {
          # "drive back/ stop intake"
          n215 = call <vilib>:"WPI_MotorControlSetOutput.vi"("Output"=0.0, "MotorControlDevRef"=w492) -> ()  [unwired: 7 in, 3 out]
          n216 = call-poly <vilib>:"WPI_RobotDriveArcadeDrive.vi"("Y axis value"=0.75, "X axis value"=0.0, "RobotDriveDevRef"=w495) -> ("RobotDriveDevRef"=w490:T10)  [unwired: 6 in, 2 out]
        }
        frame #10 {
          n217 = Wait (ms)(milliseconds to wait=u32 3000) -> ()  [unwired: 1 out]
        }
        frame #11 {
          # "stop driving/\nstart shooter"
          n218 = call <vilib>:"WPI_MotorControlSetOutput.vi"("Output"=0.3, "MotorControlDevRef"=w502) -> ()  [unwired: 7 in, 3 out]
          n219 = call-poly <vilib>:"WPI_RobotDriveArcadeDrive.vi"("Y axis value"=0.0, "X axis value"=0.0, "RobotDriveDevRef"=w505) -> ()  [unwired: 6 in, 3 out]
        }
        frame #12 {
          n220 = Wait (ms)(milliseconds to wait=u32 1000) -> ()  [unwired: 1 out]
        }
        frame #13 {
          # "start loader"
          n221 = call <vilib>:"WPI_MotorControlSetOutput.vi"("Output"=0.5, "MotorControlDevRef"=w509) -> ()  [unwired: 7 in, 3 out]
        }
        frame #14 {
          n222 = Wait (ms)(milliseconds to wait=u32 4000) -> ()  [unwired: 1 out]
        }
      }
    }
    frame "Auto 8" {
      n223 = call <vilib>:"WPI_MotorControlRefNum Registry Get.vi"("refnum name"="intake motor") -> ("MotorControlDevRef"=w516:T5)  [unwired: 9 in, 1 out]
      n224 = call <vilib>:"WPI_RobotDriveRefNum Registry Get.vi"("refnum name"="Left and Right Motors") -> ("RobotDriveDevRef"=w518:T10)  [unwired: 9 in, 1 out]
      n225 = call <vilib>:"WPI_MotorControlRefNum Registry Get.vi"("refnum name"="loader motor") -> ("MotorControlDevRef"=w511:T5)  [unwired: 9 in, 1 out]
      n226 = call <vilib>:"WPI_MotorControlRefNum Registry Get.vi"("refnum name"="shooter motor") -> ("MotorControlDevRef"=w512:T5)  [unwired: 9 in, 1 out]
      n227 = call <vilib>:"WPI_MotorControlSetOutput.vi"("Output"=0.5, "MotorControlDevRef"=w512) -> ()  [unwired: 7 in, 3 out]
      n228 = call-poly <vilib>:"WPI_RobotDriveArcadeDrive.vi"("X axis value"=-1.0, "RobotDriveDevRef"=w518) -> ()  [unwired: 7 in, 3 out]
      n229 = call <vilib>:"WPI_MotorControlSetOutput.vi"("Output"=0.5, "MotorControlDevRef"=w516) -> ()  [unwired: 7 in, 3 out]
      n230 = call <vilib>:"WPI_MotorControlSetOutput.vi"("Output"=0.5, "MotorControlDevRef"=w511) -> ()  [unwired: 7 in, 3 out]
    }
  }
  n231 = Index Array(array=w3, index=2) -> ()  [unwired: 1 out]
  n232 = call-poly <vilib>:"NT Write Value.vi"("Numeric Array"=w3, "Name"="Joystick 0/Axes") -> ()  [unwired: 9 in, 1 out]
